vi "Check for MD5 Change.vi"(8 "error in":errorcluster, 11 "configuration file page data":T1 {"custom device ref" format="%.0x"}) -> (0 "error out":errorcluster, 2 "MD5 change?":bool, 3 "configuration file page data out":T1 {"custom device ref" format="%.0x"})   [LabVIEW 2020, in "AIM ARINC 664 System Explorer.lvlib" / "Implementation.lvlib"]
uses:
  System Explorer/Implementation/Implementation.lvlib
  System Explorer/Implementation/System Explorer/Types/Configuration File Page Data.ctl
  System Explorer/Implementation/System Explorer/Types/Path Control.ctl
  System Explorer/Implementation/System Explorer/Types/Browse Button.ctl
  <vilib>/NI VeriStand/Custom Device API/Custom Device Item Ref.ctl
  <vilib>/NI VeriStand/Custom Device API/Custom Device API.lvlib
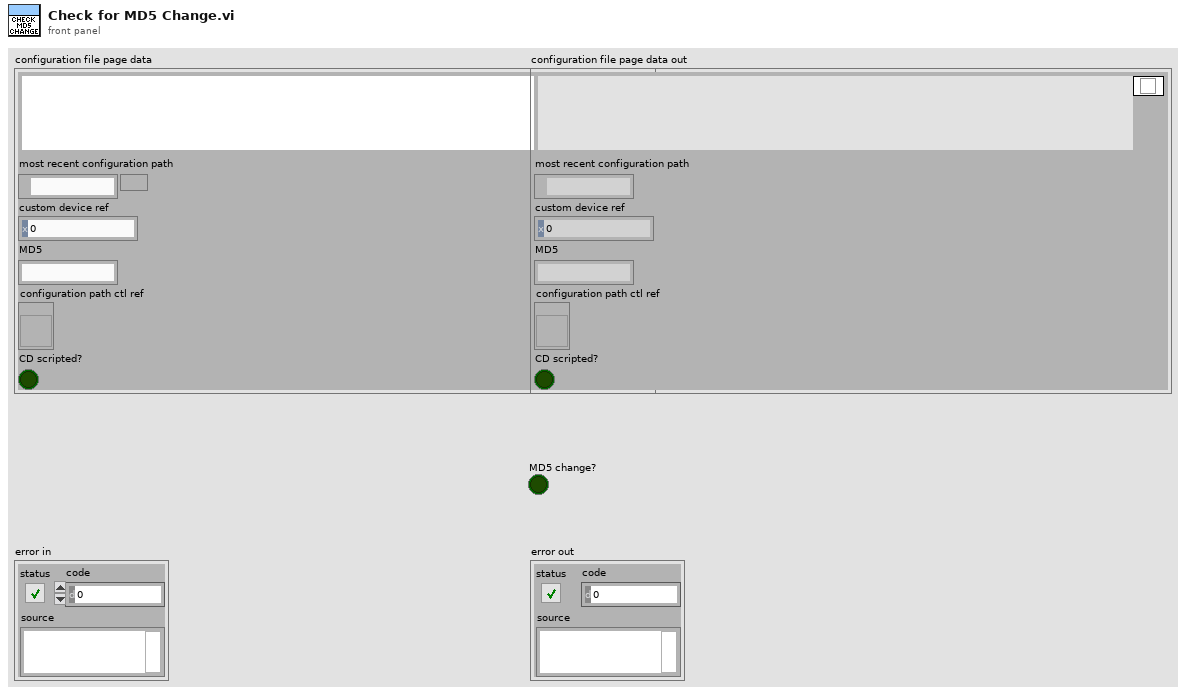
[diagram p1: front panel]
types:
  T1 = typedef "AIM ARINC 664 System Explorer.lvlib/Implementation.lvlib/Configuration File Page Data.ctl" = cluster{"Parameters":T2, "most recent configuration path":path, "custom device ref":T4, "MD5":string, "configuration path ctl ref":refnum<vi>, "CD scripted?":bool}
  T2 = typedef "AIM ARINC 664 System Explorer.lvlib/Implementation.lvlib/Path Control.ctl" = cluster{"file path":path, "Browse":T3}
  T3 = typedef "AIM ARINC 664 System Explorer.lvlib/Implementation.lvlib/Browse Button.ctl" = bool
  T4 = typedef "Custom Device API.lvlib/Custom Device Item Ref.ctl" = u64
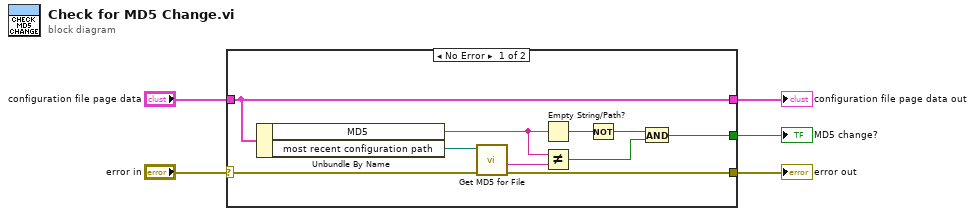
[diagram p0: block diagram]
diagram:
  n1 = case shown="No Error" "error in" {
    selector: "error in" -> [w15 w16]
    tunnel: "configuration file page data" -> [w14 w17]
    tunnel: [w14 w17] -> w3
    tunnel: [w13 w16] -> w2
    tunnel: [w6 _] -> w1
    frame No Error {
      n2 = Unbundle By Name(w14) -> ("MD5"=w10:string, "most recent configuration path"=w12:path)
      n3 = call "Get MD5 for File.vi"("error in"=w15, "Path"=w12) -> ("error out"=w13:errorcluster, "MD5"=w11:string)  [unwired: 8 in]
      n4 = Empty String/Path?(string/path=w10) -> (empty?=w9:bool)
      n5 = Not Equal?(x=w10, y=w11) -> (x != y?=w7:bool)
      n6 = Not(x=w9) -> (.not. x?=w8:bool)
      n7 = And(x=w8, y=w7) -> (x .and. y?=w6:bool)
    }
    frame Error {
    }
  }
  "configuration file page data out" <- w3
  "error out" <- w2
  "MD5 change?" <- w1
